vi "2024_day04.vi"() -> ()   [LabVIEW 2023]
uses:
  <userlib>/_OpenG.lib/string/string.llb/openg_string.lvlib
panel:
  out "Result - Task 2":i32
  out "Result - Task 1":i32
  in  "Switch":bool caption="Ex. Data  vs.  User Data"
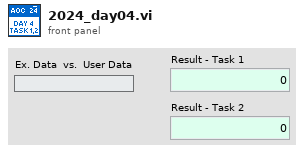
[diagram p1: front panel]
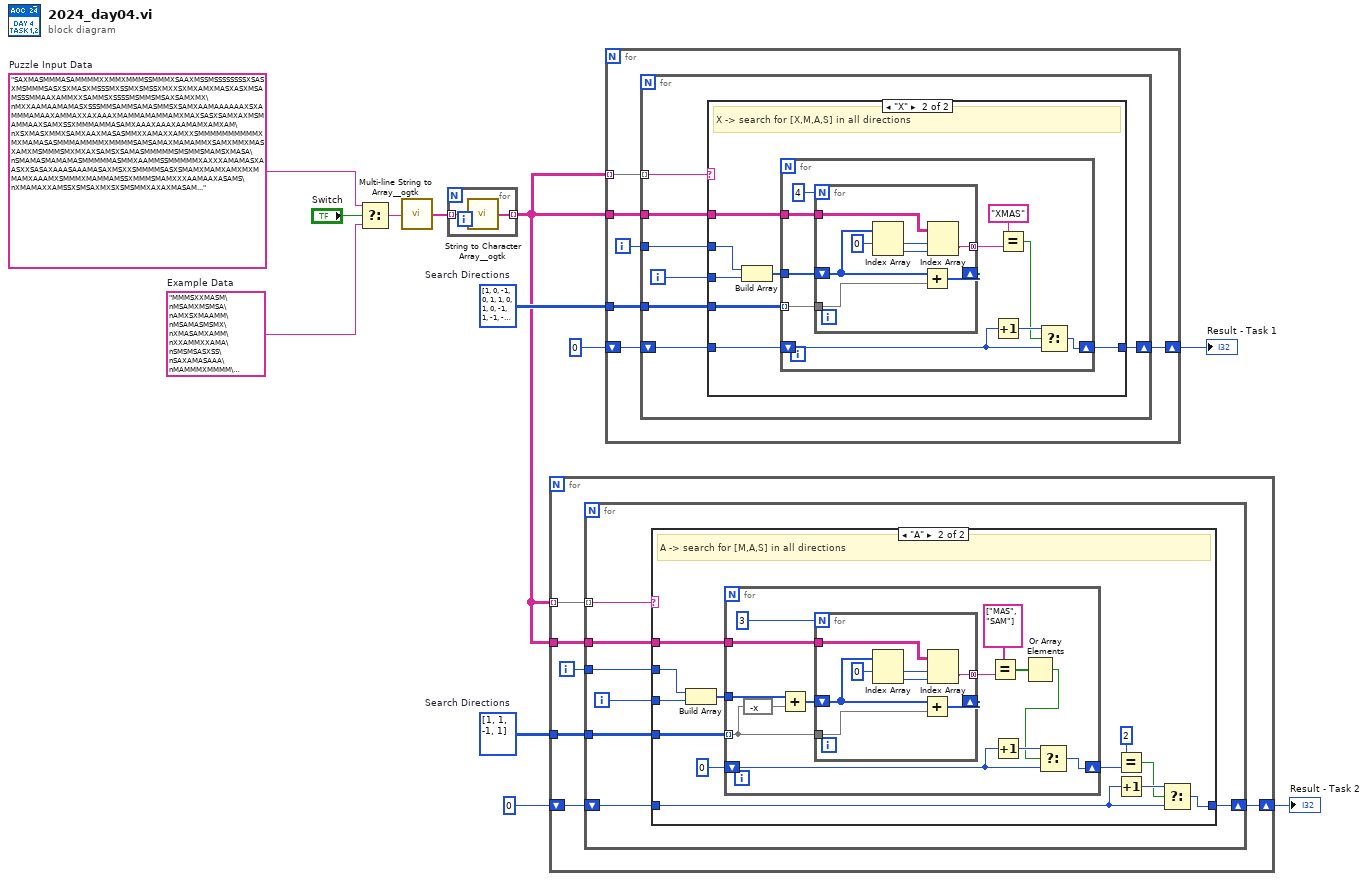
[diagram p0: block diagram]
diagram:
  w6 = i32[][] [[1, 1], [-1, 1]]  # Search Directions
  w7 = i32[][] [[1, 0], [-1, 0], [1, 1], [0, 1], [0, -1], [1, -1], [-1, 1], [-1, -1]]  # Search Directions
  w10 = "SAXMASMMMASAMMMMXXMMXMMMSSMMMXSAAXMSSMSSSSSSSSXSASXMSMMMSASXSXMASXMSSSMXSSMXSMSSXMXXSXMXAMXMASXASXMSAMSSSMMAAXAMMXXSAMMSXSSSSMSMMSMSAXSAMXMX\nMXXAAMAAMAMASXSSSMMSAMMSAMASMMSXSAMXAAMAAAAAAXSXAMMMAMAAXAMMAXXAXAAAXMAMMAMAMMAMXMAXSASXSAMXAXMSMAMMAAXSAMXSSXMMMAMMASAMXAAAXAAAXAAMAMXAMXAM\nXSXMASXMMXSAMXAAXMASASMMXXAMAXXAMXXSMMMMMMMMMMXMXMAMASASMMMAMMMMXMMMMSAMSAMAXMAMAMMXSAMXMMXMASXAMXMSMMMSMXMXAXSAMSXSAMASMMMMMSMSMMSMAMSXMASA\nSMAMASMAMAMASMMMMMASMMXAAMMSSMMMMMXAXXXAMAMASXAASXXSASAXAAASAAAMASAXMSXXSMMMMSASXSMAMXMAMXAMXMXMMAMXAAAMXSMMMXMAMMAMSSXMMMSMAMXXXAAMAAXASAMS\nXMAMAXXAMSSXSMSAXMXSXSMSMMXAXAXMASAM..."  # Puzzle Input Data
  w11 = "MMMSXXMASM\nMSAMXMSMSA\nAMXSXMAAMM\nMSAMASMSMX\nXMASAMXAMM\nXXAMMXXAMA\nSMSMSASXSS\nSAXAMASAAA\nMAMMMXMMMM\nMXMXAXMASX"  # Example Data
  n1 = Select(t=w10, s="Switch", f=w11) -> (s? t:f=w9:string)
  n2 = call <userlib>:"Multi-line String to Array__ogtk.vi"("string"=w9) -> ("lines"=w8:string[])
  n3 = for {
    tunnel: w8 -> [w14] mode=indexing
    tunnel: [w13] -> w5 mode=indexing
    n4 = call <userlib>:"String to Character Array__ogtk.vi"("Input String"=w14) -> ("Character Array"=w13:string[])
  }
  n5 = for {
    tunnel: w5 -> [w20] mode=indexing
    tunnel: w6 -> [w18]
    tunnel: w5 -> [w17]
    shift-right: [w15] -> w3
    shift-left: 0 -> [w16]
    i -> [w19]
    n6 = for {
      tunnel: w20 -> [w27] mode=indexing
      tunnel: w19 -> [w26]
      tunnel: w18 -> [w24]
      tunnel: w17 -> [w23]
      shift-right: [w21] -> w15
      shift-left: w16 -> [w22]
      i -> [w25]
      n7 = case shown="\"A\"" w27 {
        tunnel: w26 -> [_ w38]
        tunnel: w25 -> [_ w37]
        tunnel: w24 -> [_ w40]
        tunnel: w23 -> [_ w39]
        tunnel: w22 -> [w28 w30]
        tunnel: [w28 w29] -> w21
        frame Default {
          # "Skip symbol (not X)"
        }
        frame "A" {
          # "A -> search for [M,A,S] in all directions"
          n8 = Build Array(w38, w37) -> (w36:i32[])
          n9 = for {
            tunnel: w40 -> [w47] mode=indexing
            tunnel: w39 -> [w53]
            tunnel: w36 -> [w45]
            shift-right: [w50] -> w34
            shift-left: 0 -> [w49]
            n10 = expression code="-x"(w47) -> (w44:i32[])
            n11 = Add(x=w45, y=w44) -> (x+y=w46:i32[])
            n12 = for {
              N: 3 -> [_]
              tunnel: w47 -> [w59]
              tunnel: w53 -> [w61]
              shift-right: [w60] -> _
              shift-left: w46 -> [w58]
              tunnel: [w54] -> w51 mode=concatenating
              n13 = Index Array(array=w58, index #1=0 ("index")) -> (element #1=w56:i32, element #2=w55:i32)  [unwired: 1 in]
              n14 = Add(x=w58, y=w59) -> (x+y=w60:i32[])
              n15 = Index Array(array=w61, index (row)=w56, index (col)=w55) -> (element=w54:string)
            }
            n16 = Equal?(x=string[] ["MAS", "SAM"], y=w51) -> (x = y?=w43:bool[])
            n17 = Increment(x=w49) -> (x+1=w48:i32)
            n18 = Or Array Elements(Boolean array=w43) -> (logical OR=w41:bool)
            n19 = Select(t=w48, s=w41, f=w49) -> (s? t:f=w50:i32)
          }
          n20 = Equal?(x=2, y=w34) -> (x = y?=w31:bool)
          n21 = Increment(x=w30) -> (x+1=w32:i32)
          n22 = Select(t=w32, s=w31, f=w30) -> (s? t:f=w29:i32)
        }
      }
    }
  }
  "Result - Task 2" <- w3
  n23 = for {
    tunnel: w5 -> [w67] mode=indexing
    tunnel: w7 -> [w65]
    tunnel: w5 -> [w64]
    shift-right: [w62] -> w1
    shift-left: 0 -> [w63]
    i -> [w66]
    n24 = for {
      tunnel: w67 -> [w74] mode=indexing
      tunnel: w66 -> [w73]
      tunnel: w65 -> [w71]
      tunnel: w64 -> [w70]
      shift-right: [w68] -> w62
      shift-left: w63 -> [w69]
      i -> [w72]
      n25 = case shown="\"X\"" w74 {
        tunnel: w73 -> [_ w80]
        tunnel: w72 -> [_ w79]
        tunnel: w71 -> [_ w82]
        tunnel: w70 -> [_ w81]
        tunnel: w69 -> [w75 w77]
        tunnel: [w75 w76] -> w68
        frame Default {
          # "Skip symbol (not X)"
        }
        frame "X" {
          # "X -> search for [X,M,A,S] in all directions"
          n26 = Build Array(w80, w79) -> (w78:i32[])
          n27 = for {
            tunnel: w82 -> [w92] mode=indexing
            tunnel: w81 -> [w91]
            tunnel: w78 -> [w89]
            shift-right: [w83] -> w76
            shift-left: w77 -> [w84]
            n28 = for {
              N: 4 -> [_]
              tunnel: w92 -> [w98]
              tunnel: w91 -> [w100]
              shift-right: [w99] -> _
              shift-left: w89 -> [w97]
              tunnel: [w93] -> w88 mode=concatenating
              n29 = Index Array(array=w97, index #1=0 ("index")) -> (element #1=w95:i32, element #2=w94:i32)  [unwired: 1 in]
              n30 = Add(x=w97, y=w98) -> (x+y=w99:i32[])
              n31 = Index Array(array=w100, index (row)=w95, index (col)=w94) -> (element=w93:string)
            }
            n32 = Increment(x=w84) -> (x+1=w86:i32)
            n33 = Equal?(x="XMAS", y=w88) -> (x = y?=w85:bool)
            n34 = Select(t=w86, s=w85, f=w84) -> (s? t:f=w83:i32)
          }
        }
      }
    }
  }
  "Result - Task 1" <- w1
